vi "Append Node Name to Error.vi"(10 "Node Name":string, 11 "error in (no error)":errorcluster) -> (3 "error out":errorcluster)   [LabVIEW 2016]
doc: "Adds node name to error source for easier error tracking."
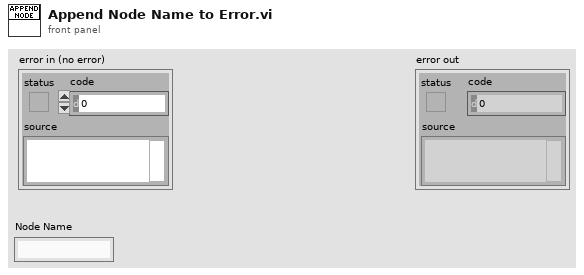
[diagram p1: front panel]
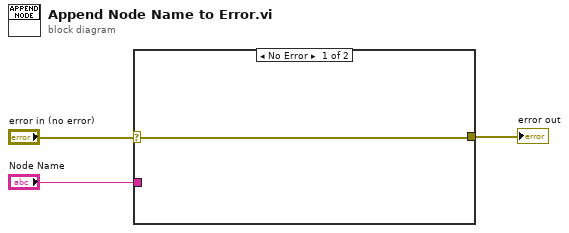
[diagram p0: block diagram]
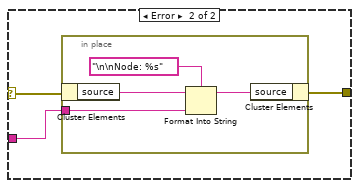
[diagram p2: hidden frame]
diagram:
  n1 = case shown="No Error" "error in (no error)" {
    selector: "error in (no error)" -> [w4 w5]
    tunnel: "Node Name" -> [_ w7]
    tunnel: [w4 w6] -> w2
    frame No Error {
    }
    frame Error {
      n2 = in-place {
        in-place-border: w7 -> [w8]
        n3 = in-place-cluster #1(w5) -> ("source"=w11:string)
        n4 = Format Into String(format string="\n\nNode: %s", initial string=w11, w8) -> (resulting string=w10:string)  [unwired: 1 in, 1 out]
        n5 = in-place-cluster #1("source"=w10) -> (w6:errorcluster)
      }
    }
  }
  "error out" <- w2
